vi "Configure Limit Test Dual Template.vi"(7 "Horizontal Division (0.0 mdiv)":dbl, 8 "error in (no error)":errorcluster, 9 "Vertical Division (0.0 mdiv)":dbl, 10 "Source (0:Channel 1)":i32(ring) items=["Channel 1"=0, "Channel 2"=1, "Math"=4], 11 "VISA resource name":refnum<visa-resource-name>) -> (0 "error out":errorcluster, 3 "VISA resource name out":refnum<visa-resource-name>)   [LabVIEW 2012, in "Tektronix TDS 200 1000 2000 Series.lvlib"]
doc: "This VI configures the settings for a limit test dual template.\n\n<b>Note(s):</b>\n1. This VI is only applicable for TBS1000B series models.\n2. This VI does not check the instrument status."
uses:
  <instrlib>/Tektronix TDS 200 1000 2000 Series/Tektronix TDS 200 1000 2000 Series.lvlib
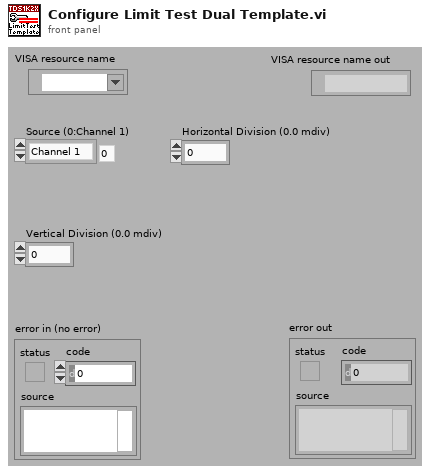
[diagram p1: front panel]
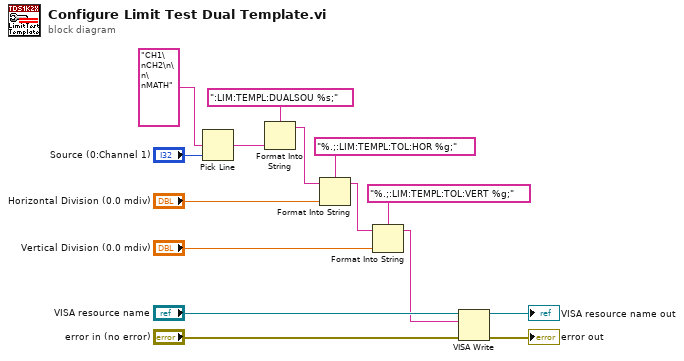
[diagram p0: block diagram]
diagram:
  n1 = Pick Line(multi-line string="CH1\nCH2\n\n\nMATH", line index="Source (0:Channel 1)") -> (output string=w11:string)  [unwired: 1 out]
  n2 = Format Into String(format string=":LIM:TEMPL:DUALSOU %s;", w11) -> (resulting string=w10:string)  [unwired: 2 in, 1 out]
  n3 = Format Into String(format string="%.;:LIM:TEMPL:TOL:HOR %g;", initial string=w10, "Horizontal Division (0.0 mdiv)") -> (resulting string=w8:string)  [unwired: 1 in, 1 out]
  n4 = Format Into String(format string="%.;:LIM:TEMPL:TOL:VERT %g;", initial string=w8, "Vertical Division (0.0 mdiv)") -> (resulting string=w1:string)  [unwired: 1 in, 1 out]
  n5 = VISA Write(VISA resource name="VISA resource name", write buffer=w1, error in (no error)="error in (no error)") -> (VISA resource name out=→"VISA resource name out":refnum<visa-resource-name>, error out=→"error out":errorcluster)  [unwired: 1 out]
